vi "DigitalInputGetState.vi"(0 "error in (no error)":errorcluster, 3 "Device In":u64) -> (7 "error out":errorcluster, 8 "State (Numeric)":i32, 9 "State":bool, 10 "Device Out":u64)   [LabVIEW 2020, in "Phidget Digital Input.lvlib"]
doc: "${State:Header}"
uses:
  <instrlib>/Phidgets/Phidget Digital Input/Phidget Digital Input.lvlib
  <instrlib>/Phidgets/Phidget Common/Phidget Common.lvlib
  phidget22.dll
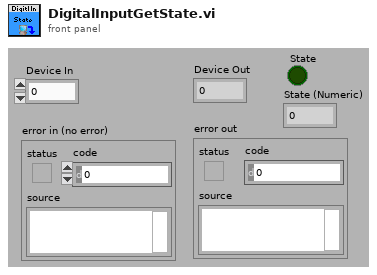
[diagram p1: front panel]
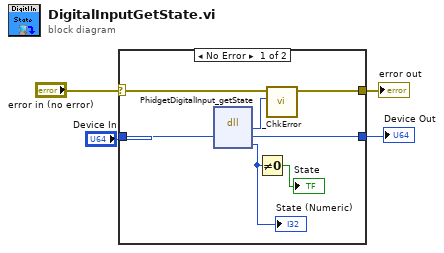
[diagram p0: block diagram]
diagram:
  n1 = case shown="No Error" "error in (no error)" {
    selector: "error in (no error)" -> [w9 w13]
    tunnel: [w8 w13] -> w3
    tunnel: "Device In" -> [w11 w12]
    tunnel: [w10 w12] -> w2
    frame No Error {
      n2 = dll-call lib="phidget22.*" fn="PhidgetDigitalInput_getState"("phid"=w11) -> ("return type"=w7:i32, "phid"=w10:u64, "state"=w5:i32)  [unwired: 4 in, 2 out]
      "State (Numeric)" <- w5
      n3 = Not Equal To 0?(x=w5) -> (x != 0?=→"State":bool)
      n4 = call <instrlib>:"_ChkError.vi"("Return Code"=w7, "error in (no error)"=w9) -> ("error out"=w8:errorcluster)  [unwired: 9 in]
    }
    frame Error {
    }
  }
  "error out" <- w3
  "Device Out" <- w2
